vi "Register gRPC Methods and Messages.vi"(8 "error in (no error)":errorcluster, 10 "gRPC ID in":T1, 11 "MeasurementServiceV1 in":refnum<class "MeasurementServiceV1.lvclass">) -> (0 "error out":errorcluster, 2 "gRPC ID out":T1, 3 "MeasurementServiceV1 out":refnum<class "MeasurementServiceV1.lvclass">)   [LabVIEW 2020, in "MeasurementLink Measurement Server.lvlib" / "MeasurementServiceV1.lvclass"]
uses:
  MeasurementServiceV1.lvclass
  <vilib>/gRPC/LabVIEW gRPC Library/Shared/grpcId.ctl
  MeasurementServiceV1.lvclass/MeasurementServiceV1.ctl
  MeasurementLink Measurement Server Internal/RPC Service/MeasurementService/MeasurementService.lvclass
  MeasurementLink Measurement Server Internal/MeasurementLink Measurement Server Internal.lvlib
  <vilib>/gRPC/LabVIEW gRPC Library/grpc-lvsupport-release.lvlib
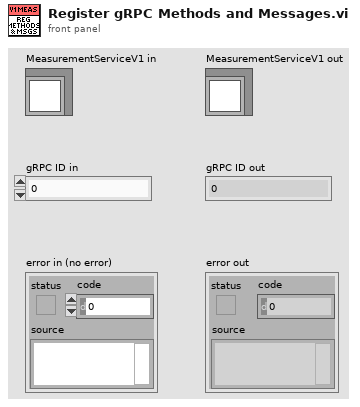
[diagram p1: front panel]
types:
  T1 = typedef "grpc-lvsupport-release.lvlib/grpcId.ctl" = u64
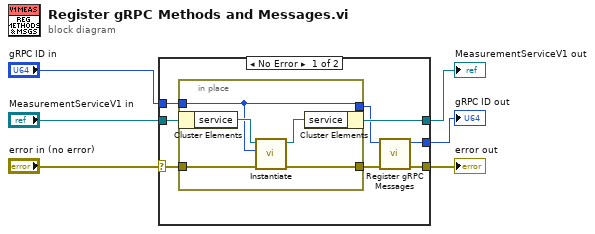
[diagram p0: block diagram]
diagram:
  n1 = case shown="No Error" "error in (no error)" {
    selector: "error in (no error)" -> [w9 w22]
    tunnel: [w13 w22] -> w5
    tunnel: [w10 w21] -> w3
    tunnel: "MeasurementServiceV1 in" -> [w11 w21]
    tunnel: "gRPC ID in" -> [w8 w20]
    tunnel: [w14 w20] -> w1
    frame No Error {
      n2 = in-place {
        in-place-border: [w17] -> w12
        in-place-border: w9 -> [w16]
        in-place-border: w8 -> [w15]
        in-place-border: [w15] -> w7
        n3 = in-place-cluster #1(w11) -> ("service"=w19:refnum<class "MeasurementService.lvclass">)
        n4 = call-dynamic "Instantiate.vi"("error in"=w16, "gRPCid"=w15, "iService"=w19) -> ("error out"=w17:errorcluster, "iService"=w18:refnum<class "MeasurementService.lvclass">)  [unwired: 7 in]
        n5 = in-place-cluster #1("service"=w18) -> (w10:refnum<class "MeasurementServiceV1.lvclass">)
      }
      n6 = call "Register gRPC Messages.vi"("error in (no error)"=w12, "gRPC ID"=w7) -> ("error out"=w13:errorcluster, "gRPC ID Out"=w14:T1)  [unwired: 8 in]
    }
    frame Error {
    }
  }
  "error out" <- w5
  "MeasurementServiceV1 out" <- w3
  "gRPC ID out" <- w1
